vi "Remove Empty and expand size 1.vi"(2 "error in (no error)":errorcluster, 3 "Data (Dictionary)":T1[](array[typedef])) -> (0 "error out":errorcluster, 1 "Array":T1[](array[typedef]))   [LabVIEW 2016]
uses:
  Data/Typedefs/Dictionary--cluster.ctl
  Data/Data.lvclass
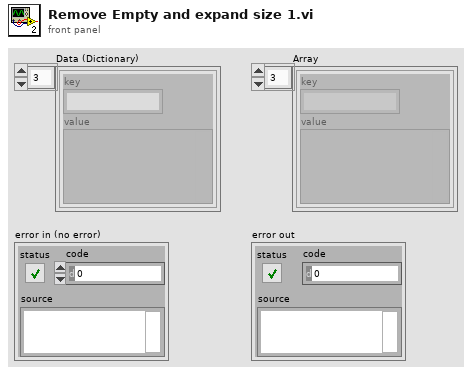
[diagram p1: front panel]
types:
  T1 = typedef "Data.lvclass/Dictionary--cluster.ctl" = cluster{"key":string, "value":variant}
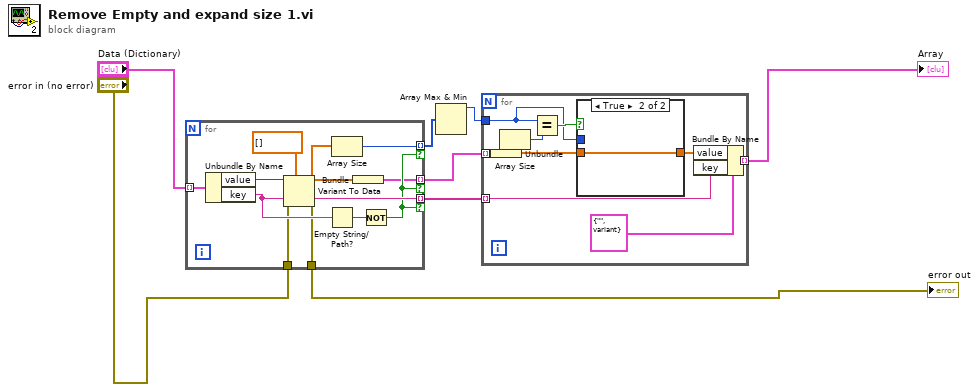
[diagram p0: block diagram]
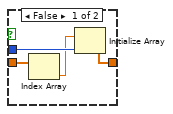
[diagram p2: hidden frame]
diagram:
  n1 = for {
    tunnel: "Data (Dictionary)" -> [w19] mode=indexing
    tunnel: [w15] -> w1 mode=indexing if=w12
    tunnel: [w9] -> w3 mode=indexing if=w12
    tunnel: [w13] -> w4 mode=indexing if=w12
    tunnel: "error in (no error)" -> [w11]
    tunnel: [w10] -> w8
    n2 = Unbundle By Name(w19) -> ("value"=w18:variant, "key"=w13:string)
    n3 = Variant To Data(error in=w11, type=dbl[] [], Variant=w18) -> (data=w14:dbl[], error out=w10:errorcluster)
    n4 = Empty String/Path?(string/path=w13) -> (empty?=w16:bool)
    n5 = Array Size(array=w14) -> (size(s)=w15:i32)
    n6 = Bundle(w14) -> (w9:cluster{dbl[]})  [unwired: 1 in]
    n7 = Not(x=w16) -> (.not. x?=w12:bool)
  }
  "error out" <- w8
  n8 = Array Max & Min(array=w1) -> (max value=w2:i32)  [unwired: 3 out]
  n9 = for {
    tunnel: w2 -> [w23]
    tunnel: w3 -> [w26] mode=indexing
    tunnel: w4 -> [w22] mode=indexing
    tunnel: [w21] -> w6 mode=indexing
    n10 = Unbundle(w26) -> (w20:dbl[])
    n11 = Array Size(array=w20) -> (size(s)=w28:i32)
    n12 = Equal?(x=w23, y=w28) -> (x = y?=w27:bool)
    n13 = case shown="True" w27 {
      tunnel: w20 -> [w32 w33]
      tunnel: [w29 w33] -> w24
      tunnel: w23 -> [w31 _]
      frame False {
        n14 = Index Array(array=w32) -> (element=w30:dbl)  [unwired: 1 in]
        n15 = Initialize Array(w30, w31) -> (w29:dbl[])
      }
      frame True {
      }
    }
    n16 = Bundle By Name(cluster=T1 {"key"="", "value"=variant} ("input cluster"), "value"=w24, "key"=w22) -> (w21:T1)
  }
  "Array" <- w6
